vi "AF_GetClassAfInfo.vi"(11 "DeriveFromClassRef":refnum<vi>) -> (0 "ClassSuffix":string, 1 "TemplateIdName":string, 2 "RootClassQualifiedName":string, 3 "AF Folder Path":path, 4 "AF Library Version":T2, 5 "ClassType":T1)   [LabVIEW 2016]
uses:
  <resource>/Framework/Providers/Open_GDS/ClassProviders/Common/AF/AF_ClassType.ctl
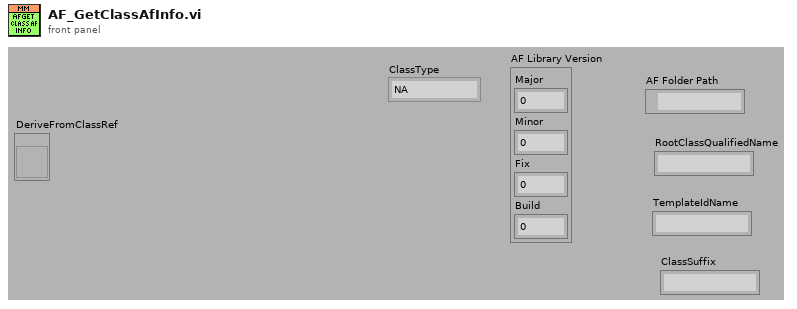
[diagram p1: front panel]
types:
  T1 = typedef "AF_ClassType.ctl" = enum16{"NA", "Actor", "Message"}
  T2 = cluster{"Major":u16, "Minor":u16, "Fix":u16, "Build":u16}
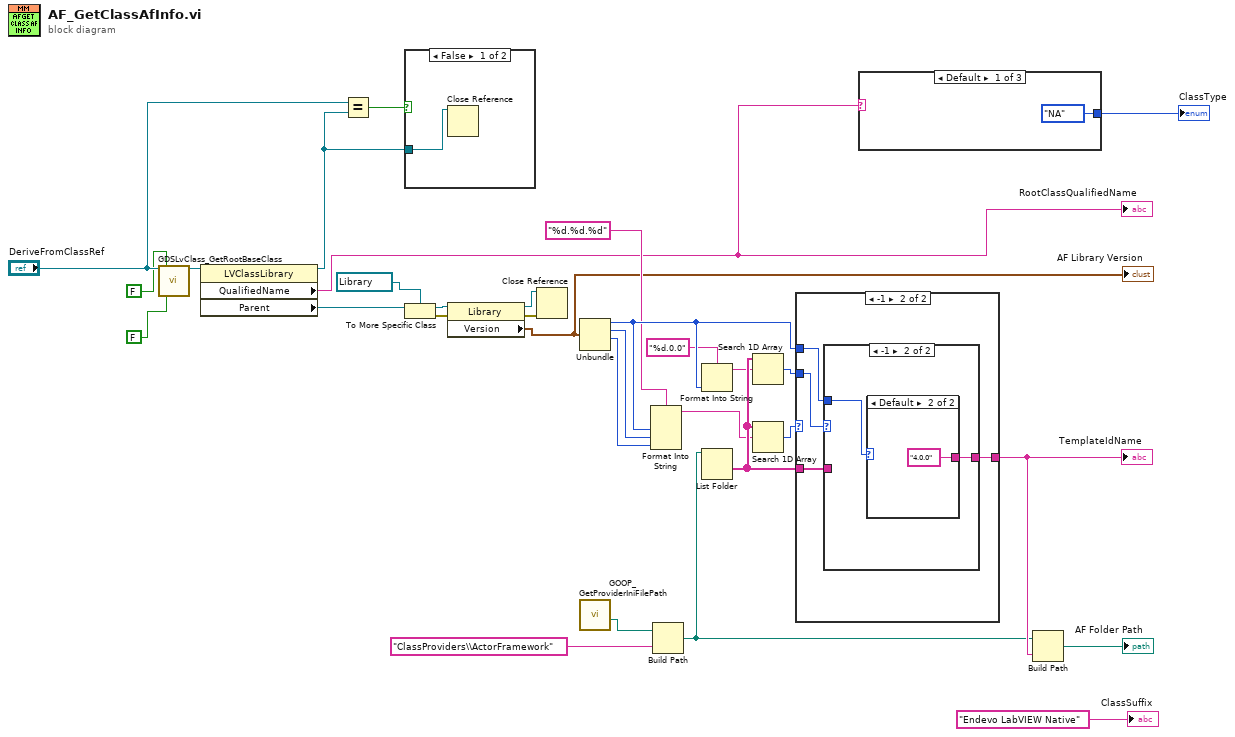
[diagram p0: block diagram]
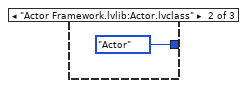
[diagram p2: hidden frame]
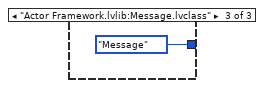
[diagram p3: hidden frame]
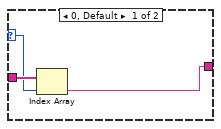
[diagram p4: hidden frame]
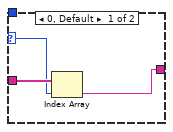
[diagram p5: hidden frame]
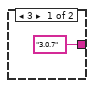
[diagram p6: hidden frame]
diagram:
  n1 = call <resource>:"GDSLvClass_GetRootBaseClass.vi"("ViRef/Path,LvClassRef/Path"="DeriveFromClassRef", "Don'tOpenReference"=FALSE, "LimitToSpecificProviderTypeOfSameType(True)"=FALSE) -> ("RootBaseClassRef"=w4:refnum<vi>)  [unwired: 11 in, 5 out]
  n2 = property class="LVClassLibrary"(reference=w4) -> (reference out=w7:refnum<vi>, "QualifiedName"=w2:string, "Parent"=w8:refnum<vi>)  [unwired: 1 in, 1 out]
  "RootClassQualifiedName" <- w2
  n3 = Equal?(x="DeriveFromClassRef", y=w7) -> (x = y?=w6:bool)
  n4 = case shown="False" w6 {
    tunnel: w7 -> [w32 _]
    frame False {
      n5 = Close Reference(reference=w32) -> ()  [unwired: 1 in, 1 out]
    }
    frame True {
    }
  }
  n6 = To More Specific Class(target class=refnum<vi> refnum ("reference"), reference=w8) -> (specific class reference=w11:refnum<vi>, error out=w10:errorcluster)  [unwired: 1 in]
  n7 = property class="Library"(reference=w11, error in=w10) -> (reference out=w12:refnum<vi>, error out=w13:errorcluster, "Version"=w14:T2)
  "AF Library Version" <- w14
  n8 = Close Reference(reference=w12, error in (no error)=w13) -> ()  [unwired: 1 out]
  n9 = Unbundle(w14) -> ("Major"=w30:u16, "Minor"=w18:u16, "Fix"=w19:u16)  [unwired: 1 out]
  n10 = call <resource>:"GOOP_GetProviderIniFilePath.vi"() -> ("ProviderMainFolder"=w15:path)  [unwired: 10 in, 1 out]
  n11 = Format Into String(format string="%d.%d.%d", w30, w18, w19) -> (resulting string=w21:string)  [unwired: 2 in, 1 out]
  n12 = Build Path(base path=w15, name or relative path="ClassProviders\\ActorFramework") -> (appended path=w25:path)
  n13 = Format Into String(format string="%d.0.0", w30) -> (resulting string=w22:string)  [unwired: 2 in, 1 out]
  n14 = List Folder(path=w25) -> (folder names=w26:string[])  [unwired: 3 in, 3 out]
  n15 = Search 1D Array(1D array=w26, element=w22) -> (index of element=w24:i32)  [unwired: 1 in]
  n16 = Search 1D Array(1D array=w26, element=w21) -> (index of element=w23:i32)  [unwired: 1 in]
  n17 = case shown="-1" w23 {
    selector: w23 -> [w34 _]
    tunnel: w24 -> [_ w39]
    tunnel: [w33 w38] -> w28
    tunnel: w26 -> [w35 w37]
    tunnel: w30 -> [_ w36]
    frame 0, Default {
      n18 = Index Array(array=w35, index=w34) -> (element=w33:string)
    }
    frame -1 {
      n19 = case shown="-1" w39 {
        selector: w39 -> [w41 _]
        tunnel: [w40 w44] -> w38
        tunnel: w37 -> [w42 _]
        tunnel: w36 -> [_ w43]
        frame 0, Default {
          n20 = Index Array(array=w42, index=w41) -> (element=w40:string)
        }
        frame -1 {
          n21 = case shown="Default" w43 {
            tunnel: ["3.0.7" ("TemplateIdName") "4.0.0" ("TemplateIdName")] -> w44
            frame 3 {
            }
            frame Default {
            }
          }
        }
      }
    }
  }
  "TemplateIdName" <- w28
  n22 = case shown="Default" w2 {
    tunnel: [AF_ClassType."NA" ("ClassType") AF_ClassType."Actor" ("ClassType") AF_ClassType."Message" ("ClassType")] -> w1
    frame Default {
    }
    frame "Actor Framework.lvlib:Actor.lvclass" {
    }
    frame "Actor Framework.lvlib:Message.lvclass" {
    }
  }
  "ClassType" <- w1
  n23 = Build Path(base path=w25, name or relative path=w28) -> (appended path=→"AF Folder Path":path)
  "ClassSuffix" <- "Endevo LabVIEW Native" ("ClassSuffix")
